vi "noveno.vi"() -> ()   [LabVIEW 2012]
panel:
  out "Cluster 2":T1
  in  "Cluster":T1
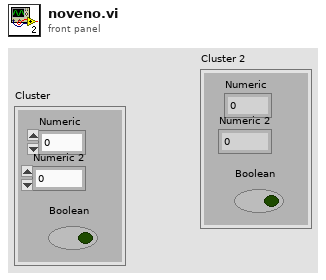
[diagram p1: front panel]
types:
  T1 = cluster{"Numeric":dbl, "Numeric 2":dbl, "Boolean":bool}
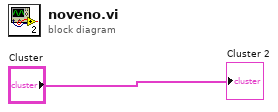
[diagram p0: block diagram]
diagram:
  "Cluster 2" <- "Cluster"
